vi "get column DBL.vi"(8 "error in":errorcluster, 10 "column index":i32, 11 "ppStmt":i64) -> (0 "error out":errorcluster, 3 "value":dbl)   [LabVIEW 2014, in "SQLite3LV.lvlib" / "cursor.lvclass"]
uses:
  cursor.lvclass
  sqlite3_64.dll
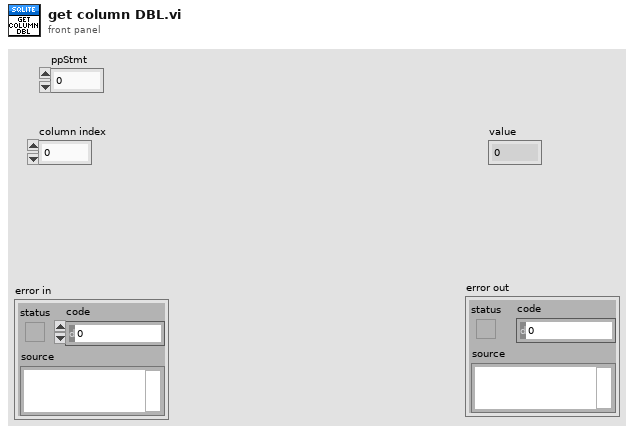
[diagram p1: front panel]
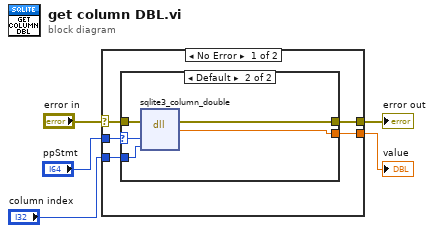
[diagram p0: block diagram]
diagram:
  n1 = case shown="No Error" "error in" {
    selector: "error in" -> [w10 w17]
    tunnel: [w8 w17] -> w2
    tunnel: [w9 _] -> w1
    tunnel: "ppStmt" -> [w7 _]
    tunnel: "column index" -> [w6 _]
    frame No Error {
      n2 = case shown="Default" w7 {
        selector: w7 -> [_ w13]
        tunnel: w10 -> [w11 w16]
        tunnel: [_ w15] -> w9
        tunnel: [w11 w14] -> w8
        tunnel: w6 -> [_ w12]
        frame 0 {
        }
        frame Default {
          n3 = dll-call lib="C:/Users/BobUser/Desktop/LVTables/sqlite3**.*" fn="sqlite3_column_double"(error in=w16, "pStmt"=w13, "iCol"=w12) -> (error out=w14:errorcluster, "value"=w15:dbl)  [unwired: 4 in, 1 out]
        }
      }
    }
    frame Error {
    }
  }
  "error out" <- w2
  "value" <- w1
